vi "Keyence LJ-X8000 Read Profiles(for High Speed Data Communication).vi"() -> ()   [LabVIEW 2014]
doc: "This example mainly indicates how to acquire profiles from controllers by using <B>Read Profiles (for High-Speed Communication)</B> VI via high-speed communication."
uses:
  Public/Clusters/Ethernet Config.ctl
  Public/Clusters/High-Speed Comm Start Req.ctl
  Public/Constants/High-Speed Comm Start Pos.ctl
  Public/Constants/High-Speed Receive Ratio.ctl
  Public/Clusters/Profile Info.ctl
  KEYENCE LJ-X8000A.lvlib
panel:
  out "数组":i32[](array[numeric])
  out "error out":errorcluster
  out "サイズ":i32[](array[numeric])
  out "Comm":bool
  out "Monitoring":bool
  out "Timeout Cnt":u32
  out "Height Image":i16[][](graph)
  out "Read Cnt":u32
  out "Notify":u32
  out "Buf Usage Rate":u32
  out "Profile Info":T1
  in  "Start Req":T2={"High-Speed Comm Start Pos"=2, "Read Profile Cnt"=1000, "High-Speed Receive Ratio"=16} {"High-Speed Receive Ratio" items=["LOWEST"=0, "LOW"=16, "MIDDLE"=17, "HIGH"=18, "HIGHEST"=32]; "High-Speed Comm Start Pos" items=["SEND COMPLETE POS", "OLDEST", "NEXT"]}
  in  "Port No":u16=24692
  in  "Stop Monitoring":bool
  in  "Start Monitoring":bool
  in  "Stop High Speed Comm":bool
  in  "Start High Speed Comm":bool
  in  "Stop VI":bool
  in  "Ethernet Config":T5={"IP Address"=[192, 168, 0, 1], "Port No"=24691}
  # "Read Profiles Start/Stop"
  # "High Speed Data Communication Start/Stop"
  # "Communication Configuration"
  # "Output from Read Profiles VI"
  # "Communication Configuration\nfor High Speed Communication"
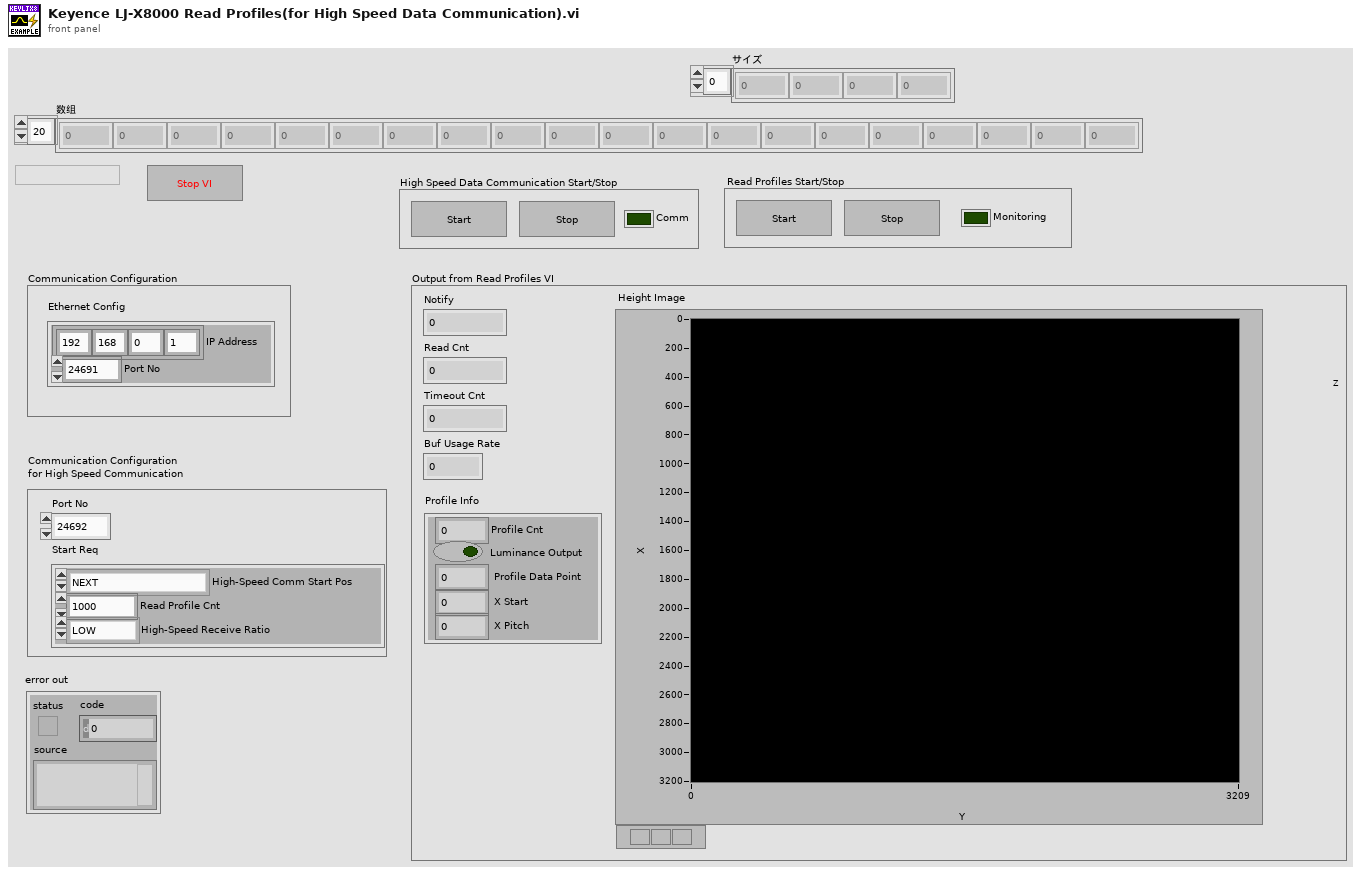
[diagram p1: front panel]
types:
  T1 = typedef "KEYENCE LJ-X8000A.lvlib/Profile Info.ctl" = cluster{"Profile Cnt":u8, "Luminance Output":bool, " Profile Data Point":u16, " X Start":i32, " X Pitch":i32}
  T2 = typedef "KEYENCE LJ-X8000A.lvlib/High-Speed Comm Start Req.ctl" = cluster{"High-Speed Comm Start Pos":T3, "Read Profile Cnt":u32, "High-Speed Receive Ratio":T4}
  T3 = typedef "KEYENCE LJ-X8000A.lvlib/High-Speed Comm Start Pos.ctl" = u8
  T4 = typedef "KEYENCE LJ-X8000A.lvlib/High-Speed Receive Ratio.ctl" = u8
  T5 = typedef "KEYENCE LJ-X8000A.lvlib/Ethernet Config.ctl" = cluster{"IP Address":u8[], "Port No":u16}
  T6 = enum8{"Enabled", "Disabled", "Disabled and Grayed Out"}
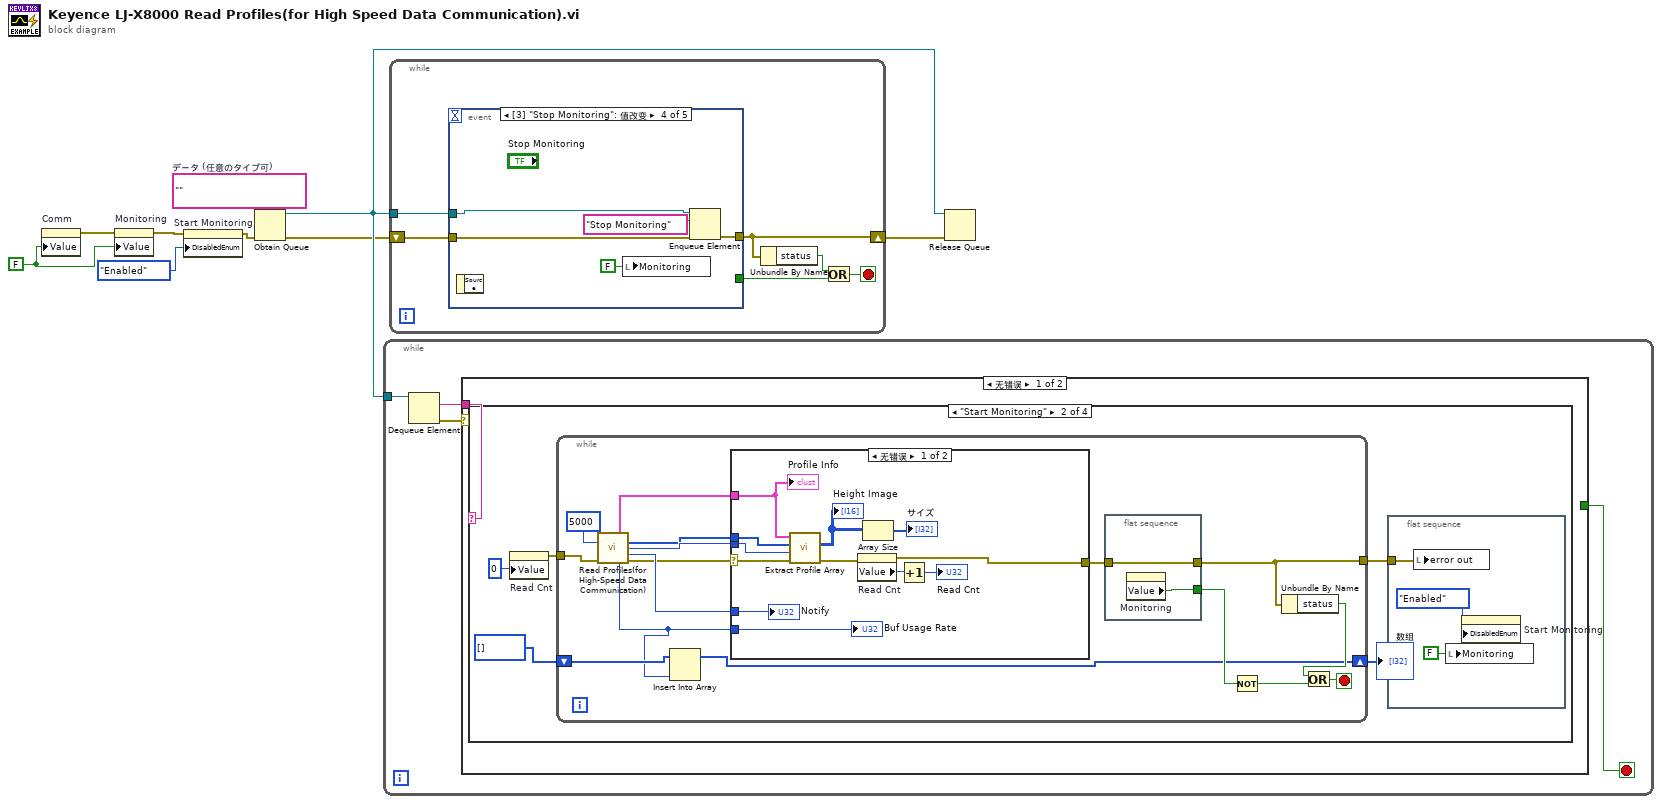
[diagram p0: block diagram]
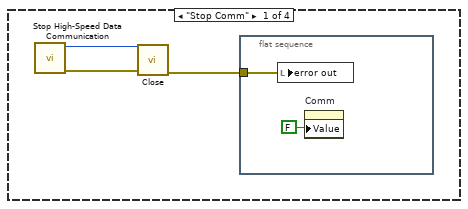
[diagram p2: hidden frame]
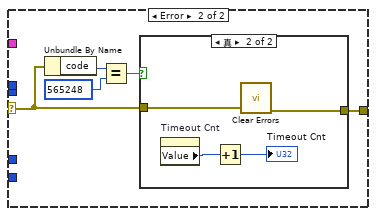
[diagram p3: hidden frame]
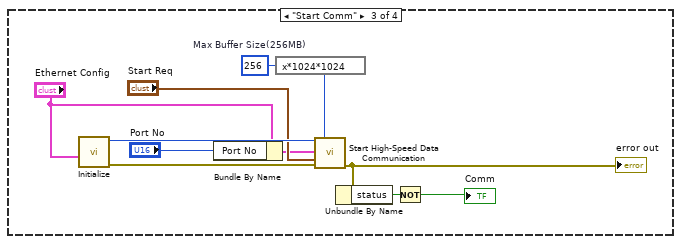
[diagram p5: hidden frame]
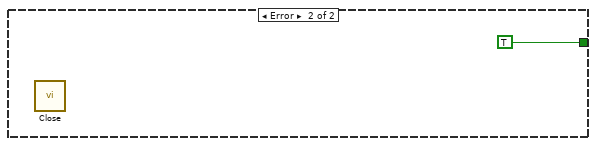
[diagram p7: hidden frame]
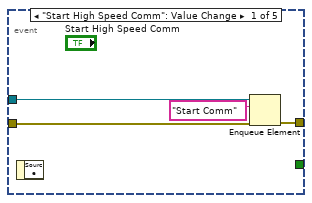
[diagram p8: hidden frame]
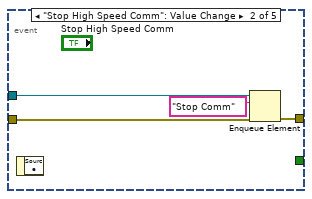
[diagram p9: hidden frame]
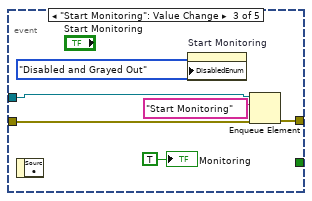
[diagram p10: hidden frame]
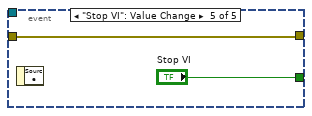
[diagram p11: hidden frame]
diagram:
  w5 = FALSE ("Monitoring")
  w7 = ""  # データ (任意のタイプ可)
  n1 = property on="Comm" class="Bool (严格)"("Value"=w5) -> (error out=w6:errorcluster)  [unwired: 2 in, 1 out]
  n2 = property on="Monitoring" class="Bool (严格)"(error in=w6, "Value"=w5) -> (error out=w4:errorcluster)  [unwired: 1 in, 1 out]
  n3 = property on="Start Monitoring" class="Bool"(error in=w4, "DisabledEnum"=T6."Enabled" ("–³Œø")) -> (error out=w2:errorcluster)  [unwired: 1 in, 1 out]
  n4 = Obtain Queue(element data type=w7, error in (no error)=w2) -> (queue out=w8:refnum<queue>, error out=w3:errorcluster)  [unwired: 3 in, 1 out]
  n5 = while {
    tunnel: w8 -> [w13]
    stop <- w10 stop-if-true
    n6 = Dequeue Element(queue=w13) -> (element=w11:string, error out=w12:errorcluster)  [unwired: 2 in, 2 out]
    n7 = case shown="无错误" w12 {
      tunnel: w11 -> [w14 _]
      tunnel: [_ TRUE] -> w10
      frame No Error {
        n8 = case shown="\"Start Monitoring\"" w14 {
          frame "Stop Comm" {
            n9 = call "Stop High-Speed Data Communication.vi"() -> ("error out"=w17:errorcluster, "Device ID out"=w16:i32)  [unwired: 10 in]
            n10 = call "Close.vi"("error in (no error)"=w17, "Device ID (0)"=w16) -> ("error out"=w15:errorcluster)  [unwired: 8 in, 1 out]
            n11 = flat-sequence {
              tunnel: w15 -> [w19]
              frame #0 {
                n12 = local write "error out"(w19) -> ()
                n13 = property on="Comm" class="Bool (严格)"("Value"=FALSE ("Comm")) -> ()  [unwired: 2 in, 2 out]
              }
            }
          }
          frame "Start Monitoring" {
            n14 = property on="Read Cnt" class="DigNum (严格)"("Value"=u32 0 ("Read Cnt")) -> (error out=w23:errorcluster)  [unwired: 2 in, 1 out]
            n15 = while {
              tunnel: w23 -> [w39]
              tunnel: [w34] -> w24
              shift-right: [w28] -> w20
              shift-left: i32[] [] -> [w30]
              stop <- w36 stop-if-true
              n16 = call "Read Profiles(for High-Speed Data Communication).vi"("Timeout"=u32 5000, "error in (no error)"=w39) -> ("Profile Info"=w43:T1, "Profile Data"=w37:u32[], "Rsp Profile Cnt"=w40:u32, "Notify"=w41:u32, "Buf Usage Rate"=w29:u32, "error out"=w32:errorcluster)  [unwired: 7 in, 1 out]
              n17 = Insert Into Array(array=w30, new element=w29) -> (w28:i32[])  [unwired: 1 in]
              n18 = case shown="无错误" w32 {
                selector: w32 -> [w52 w62]
                tunnel: w29 -> [w57 _]
                tunnel: w43 -> [w51 _]
                tunnel: w41 -> [w56 _]
                tunnel: w40 -> [w49 _]
                tunnel: [w53 w61] -> w35
                tunnel: w37 -> [w50 _]
                frame No Error {
                  n19 = call "Extract Profile Array.vi"("error in (no error)"=w52, "Profile Cnt"=w49, "Profile Data"=w50, "Profile Info"=w51) -> ("error out"=w48:errorcluster, "16位forImage"=w47:i16[][])  [unwired: 4 in, 2 out]
                  "Height Image" <- w47
                  n20 = property on="Read Cnt" class="DigNum (严格)"(error in=w48) -> (error out=w53:errorcluster, "Value"=w55:u32)  [unwired: 1 in, 1 out]
                  n21 = Array Size(array=w47) -> (size(s)=→"サイズ":i32[])
                  n22 = Increment(x=w55) -> (x+1=→"Read Cnt":u32)
                  "Buf Usage Rate" <- w57
                  "Profile Info" <- w51
                  "Notify" <- w56
                }
                frame Error {
                  n23 = Unbundle By Name(w62) -> ("code"=w60:i32)
                  n24 = Equal?(x=w60, y=565248) -> (x = y?=w58:bool)
                  n25 = case shown="真" w58 {
                    tunnel: w62 -> [w63 w67]
                    tunnel: [w63 w66] -> w61
                    frame False {
                    }
                    frame True {
                      n26 = property on="Timeout Cnt" class="DigNum (严格)"() -> ("Value"=w65:u32)  [unwired: 2 in, 2 out]
                      n27 = Increment(x=w65) -> (x+1=→"Timeout Cnt":u32)
                      n28 = call <vilib>:"Clear Errors.vi"("error in (no error)"=w67) -> ("error out"=w66:errorcluster)  [unwired: 5 in, 1 out]
                    }
                  }
                }
              }
              n29 = flat-sequence {
                tunnel: w35 -> [w45]
                tunnel: [w45] -> w34
                tunnel: [w44] -> w33
                frame #0 {
                  n30 = property on="Monitoring" class="Bool (严格)"() -> ("Value"=w44:bool)  [unwired: 2 in, 2 out]
                }
              }
              n31 = Not(x=w33) -> (.not. x?=w38:bool)
              n32 = Unbundle By Name(w34) -> ("status"=w31:bool)
              n33 = Or(x=w31, y=w38) -> (x .or. y?=w36:bool)
            }
            "数组" <- w20
            n34 = flat-sequence {
              tunnel: w24 -> [w25]
              frame #0 {
                n35 = local write "error out"(w25) -> ()
                n36 = local write "Monitoring"(FALSE ("Monitoring")) -> ()
                n37 = property on="Start Monitoring" class="Bool"("DisabledEnum"=T6."Enabled" ("–³Œø")) -> ()  [unwired: 2 in, 2 out]
              }
            }
          }
          frame "Start Comm" {
            w69 = u32 256  # Max Buffer Size(256MB)
            n38 = call "Initialize.vi"("Ethernet Config"="Ethernet Config") -> ("error out"=w71:errorcluster, "Device ID out"=w78:i32)  [unwired: 9 in]
            n39 = Bundle By Name(cluster="Ethernet Config", "Port No"="Port No") -> (w74:T5)
            n40 = expression code="x*1024*1024"(w69) -> (w73:u32)
            n41 = call "Start High-Speed Data Communication.vi"("Device ID"=w78, "Max Buffer Size"=w73, "Ethernet Config"=w74, "Start Req"="Start Req", "error in (no error)"=w71) -> ("error out"=w70:errorcluster)  [unwired: 9 in, 1 out]
            "error out" <- w70
            n42 = Unbundle By Name(w70) -> ("status"=w68:bool)
            n43 = Not(x=w68) -> (.not. x?=→"Comm":bool)
          }
          frame Default {
          }
        }
      }
      frame Error {
        n44 = call "Close.vi"() -> ()  [unwired: 10 in, 2 out]
      }
    }
  }
  n45 = while {
    shift-right: [w81] -> w9
    shift-left: w3 -> [w84]
    tunnel: w8 -> [w85]
    stop <- w82 stop-if-true
    n46 = event shown="[3] \"Stop Monitoring\": 值改变" {
      selector: _ -> [_ _ _ _ _]
      dyn-events: _ -> [_ _ _ _ _]
      timeout: _ -> [_ _ _ _ _]
      tunnel: w85 -> [w89 w93 w95 w100 _]
      tunnel: w84 -> [w88 w92 w99 w104 w106]
      tunnel: [w87 w91 w98 w103 w106] -> w81
      tunnel: [_ _ _ _ "Stop VI"] -> w83
      event "Start High Speed Comm": Value Change {
        n47 = event-data() -> ()  [unwired: 1 in, 1 out]
        n48 = Enqueue Element(queue=w89, element="Start Comm", error in (no error)=w88) -> (error out=w87:errorcluster)  [unwired: 1 in, 2 out]
      }
      event "Stop High Speed Comm": Value Change {
        n49 = event-data() -> ()  [unwired: 1 in, 1 out]
        n50 = Enqueue Element(queue=w93, element="Stop Comm", error in (no error)=w92) -> (error out=w91:errorcluster)  [unwired: 1 in, 2 out]
      }
      event "Start Monitoring": Value Change {
        n51 = event-data() -> ()  [unwired: 1 in, 1 out]
        n52 = property on="Start Monitoring" class="Bool"("DisabledEnum"=T6."Disabled and Grayed Out" ("–³Œø")) -> ()  [unwired: 2 in, 2 out]
        n53 = Enqueue Element(queue=w95, element="Start Monitoring", error in (no error)=w99) -> (error out=w98:errorcluster)  [unwired: 1 in, 2 out]
        "Monitoring" <- TRUE ("Monitoring")
      }
      event "Stop Monitoring": Value Change {
        n54 = event-data() -> ()  [unwired: 1 in, 1 out]
        n55 = local write "Monitoring"(FALSE ("Monitoring")) -> ()
        n56 = Enqueue Element(queue=w100, element="Stop Monitoring", error in (no error)=w104) -> (error out=w103:errorcluster)  [unwired: 1 in, 2 out]
      }
      event "Stop VI": Value Change {
        n57 = event-data() -> ()  [unwired: 1 in, 1 out]
      }
    }
    n58 = Unbundle By Name(w81) -> ("status"=w80:bool)
    n59 = Or(x=w80, y=w83) -> (x .or. y?=w82:bool)
  }
  n60 = Release Queue(queue=w8, error in (no error)=w9) -> ()  [unwired: 1 in, 3 out]
